vi "search house.vi"(8 "Nr Türen":i32, 9 "Häuser koord":i32[][](array[numeric])=[[160, 0], [220, 0], [220, 0], [280, 0], [280, 0], [340, 0], [20, 20], [80, 20], [190, 20], [250, 20], [310, 20], [220, 40], [280, 40], [50, 40], [120, 40], [160, 40], [220, 40], [280, 40], [340, 40], [340, 40], [160, 40], [380, 40], [20, 60], [80, 60], [140, 70], [360, 70], [160, 100], [380, 100], [120, 100], [120, 100], [180, 100], [240, 100], [340, 100], [380, 100], [280, 100], [320, 100], [20, 120], [60, 120], [150, 120], [350, 120], [260, 130], [180, 140], [120, 140], [320, 140], [320, 140], [380, 140], [360, 140], [40, 150], [280, 160], [240, 160], [340, 170], [20, 180], [60, 180], [45, 180], [5, 180], [360, 200], [160, 200], [320, 200], [120, 200], [25, 210], [200, 220], [240, 220], [140, 230], [5, 240], [0, 240], [45, 240], [60, 240], [220, 250], [120, 260], [30, 260], [130, 260], [160, 260], [190, 260], [60, 280], [200, 280], [240, 280], [0, 280], [160, 280], [300, 280], [360, 280], [240, 290], [200, 290], [130, 300], [190, 300], [330, 300], [220, 320], [300, 320], [360, 320], [300, 320], [360, 320], [330, 340], [200, 350], [240, 350], [300, 360], [360, 360], [30, 400], [90, 400], [60, 420], [30, 440], [90, 440]], 10 "Türen":string[][](array[string])=[["250", "40"], ["310", "40"], ["50", "60"], ["120", "70"], ["340", "70"], ["40", "120"], ["180", "120"], ["320", "120"], ["240", "130"], ["320", "170"], ["45", "210"], ["220", "220"], ["160", "230"], ["60", "260"], ["330", "280"], ["160", "300"], ["240", "320"], ["330", "360"], ["60", "400"], ["190", "40"]], 11 "Häuserlagen":cluster{i32[][]}[](array[cluster])=[{[[-30, 0], [30, 0], [30, -40], [-30, -40], [0, -20]]}, {[[0, 30], [0, -30], [-40, -30], [-40, 30], [-20, 0]]}, {[[30, 0], [-30, 0], [-30, 40], [30, 40], [0, 20]]}, {[[0, -30], [0, 30], [40, 30], [40, -30], [20, 0]]}, {[[0, 20], [60, 20], [60, -20], [0, -20], [30, 0]]}, {[[20, 0], [20, -60], [-20, -60], [-20, 0], [0, -30]]}, {[[0, -20], [-60, -20], [-60, 20], [0, 20], [-30, 0]]}, {[[-20, 0], [-20, 60], [20, 60], [20, 0], [0, 30]]}]) -> (3 "Häuser":T1[](array[typedef]))   [LabVIEW 2019]
uses:
  Haus.ctl
  Koordinate.ctl
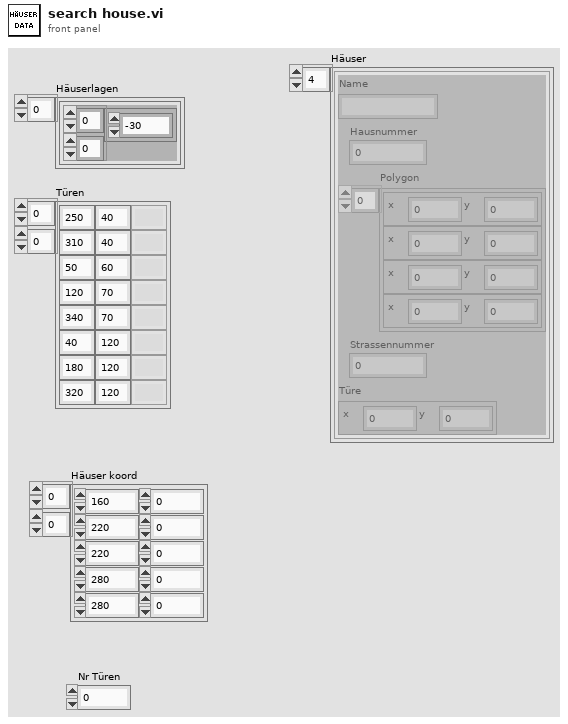
[diagram p1: front panel]
types:
  T1 = typedef "Haus.ctl" = cluster{"Name":string, "Hausnummer":u8, "Polygon":T2[], "Strassennummer":u8, "Türe":T2}
  T2 = typedef "Koordinate.ctl" = cluster{"x":dbl, "y":dbl}
  T3 = cluster{"Häuser koord[0]":i32, "Häuser koord[1]":i32}
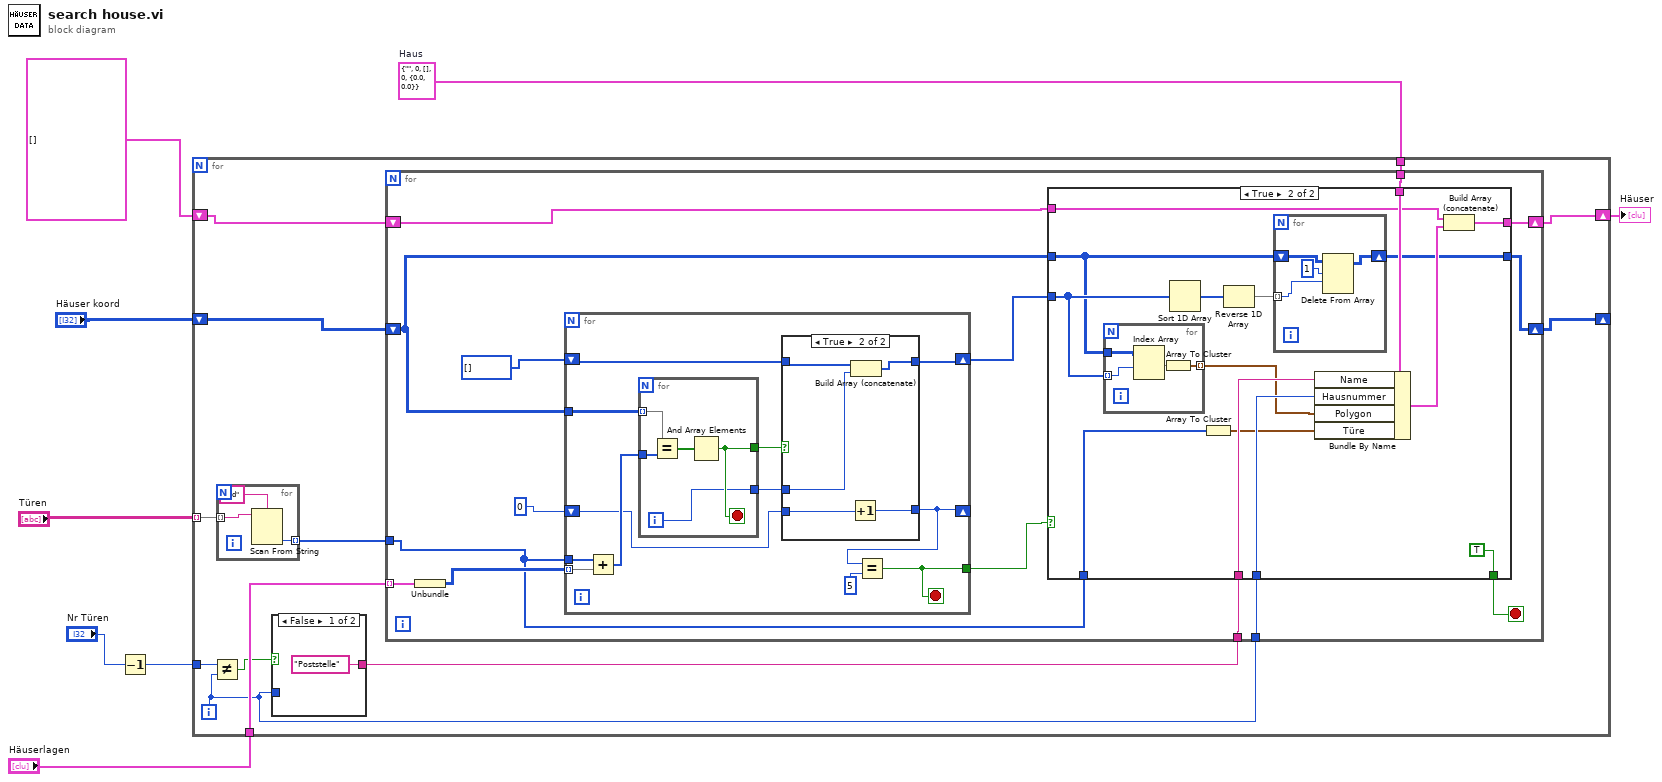
[diagram p0: block diagram]
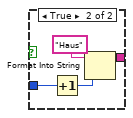
[diagram p2: hidden frame]
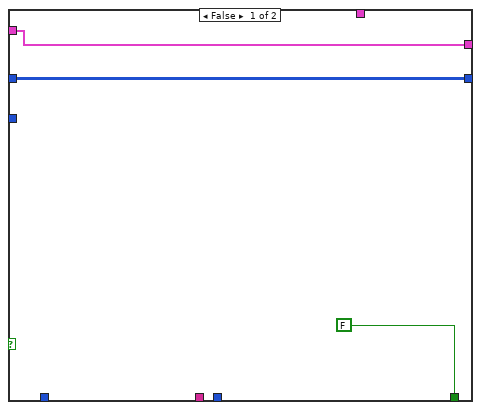
[diagram p4: hidden frame]
diagram:
  w5 = T1 {"Name"="", "Hausnummer"=0, "Polygon"=[], "Strassennummer"=0, "Türe"={"x"=0.0, "y"=0.0}}  # Haus
  n1 = Decrement(x="Nr Türen") -> (x-1=w1:i32)
  n2 = for {
    tunnel: "Türen" -> [w20] mode=indexing
    shift-right: [w13] -> _
    shift-left: "Häuser koord" -> [w18]
    tunnel: "Häuserlagen" -> [w19]
    shift-right: [w12] -> w4
    shift-left: T1[] [] -> [w15]
    tunnel: w5 -> [w16]
    tunnel: w1 -> [w11]
    i -> [w10]
    n3 = Not Equal?(x=w11, y=w10) -> (x != y?=w9:bool)
    n4 = for {
      tunnel: w20 -> [w93] mode=indexing
      tunnel: [w91] -> w17 mode=indexing
      n5 = Scan From String(format string="%d", input string=w93) -> (output 1=w91:i32)  [unwired: 3 in, 3 out]
    }
    n6 = case shown="False" w9 {
      tunnel: ["Poststelle" w25] -> w14
      tunnel: w10 -> [_ w23]
      frame False {
      }
      frame True {
        n7 = Increment(x=w23) -> (x+1=w24:i32)
        n8 = Format Into String(initial string="Haus", w24) -> (resulting string=w25:string)  [unwired: 2 in, 1 out]
      }
    }
    n9 = for {
      tunnel: w19 -> [w40] mode=indexing
      shift-right: [w27] -> w13
      shift-left: w18 -> [w28]
      tunnel: w17 -> [w38]
      tunnel: w16 -> [w37]
      shift-right: [w29] -> w12
      shift-left: w15 -> [w36]
      tunnel: w14 -> [w35]
      tunnel: w10 -> [w34]
      stop <- w31 stop-if-true
      n10 = Unbundle(w40) -> (w39:i32[][])
      n11 = for {
        tunnel: w39 -> [w52] mode=indexing
        tunnel: w38 -> [w49]
        shift-right: [w45] -> w30
        shift-left: i32[] [] -> [w47]
        shift-right: [w42] -> _
        shift-left: 0 -> [w46]
        tunnel: w28 -> [w51]
        tunnel: [w41] -> w26
        stop <- w41 stop-if-true
        n12 = Add(x=w49, y=w52) -> (x+y=w50:i32[])
        n13 = for {
          tunnel: w51 -> [w63] mode=indexing
          tunnel: w50 -> [w64]
          tunnel: [w61] -> w44
          tunnel: [w60] -> w48
          i -> [w60]
          stop <- w61 stop-if-true
          n14 = Equal?(x=w63, y=w64) -> (x = y?=w62:bool[])
          n15 = And Array Elements(Boolean array=w62) -> (logical AND=w61:bool)
        }
        n16 = case shown="True" w44 {
          tunnel: w46 -> [w54 w59]
          tunnel: [w54 w58] -> w42
          tunnel: [w53 w56] -> w45
          tunnel: w47 -> [w53 w57]
          tunnel: w48 -> [_ w55]
          frame False {
          }
          frame True {
            n17 = Increment(x=w59) -> (x+1=w58:i32)
            n18 = Build Array (concatenate)(w57, w55) -> (w56:i32[])
          }
        }
        n19 = Equal?(x=w42, y=5) -> (x = y?=w41:bool)
      }
      n20 = case shown="True" w26 {
        tunnel: w37 -> [_ w82]
        tunnel: w36 -> [w66 w76]
        tunnel: w35 -> [_ w81]
        tunnel: w34 -> [_ w80]
        tunnel: w38 -> [_ w79]
        tunnel: [FALSE TRUE] -> w31
        tunnel: w30 -> [_ w70]
        tunnel: [w66 w75] -> w29
        tunnel: w28 -> [w65 w69]
        tunnel: [w65 w71] -> w27
        frame False {
        }
        frame True {
          n21 = for {
            tunnel: w70 -> [w85] mode=indexing
            tunnel: w69 -> [w86]
            tunnel: [w83] -> w68 mode=indexing
            n22 = Index Array(array=w86, index (row)=w85) -> (element=w84:i32[])  [unwired: 1 in]
            n23 = Array To Cluster(array=w84) -> (cluster=w83:T3)
          }
          n24 = Sort 1D Array(array=w70) -> (sorted array=w73:i32[])
          n25 = Array To Cluster(array=w79) -> (cluster=w78:cluster{"[0]":i32, "[1]":i32})
          n26 = Reverse 1D Array(array=w73) -> (reversed array=w72:i32[])
          n27 = for {
            shift-right: [w89] -> w71
            shift-left: w69 -> [w90]
            tunnel: w72 -> [w88] mode=indexing
            n28 = Delete From Array(array=w90, length=1, index (row)=w88) -> (array with subset deleted=w89:i32[][])  [unwired: 1 in, 1 out]
          }
          n29 = Bundle By Name(cluster=w82, "Name"=w81, "Hausnummer"=w80, "Polygon"=w68, "Türe"=w78) -> (w74:T1)
          n30 = Build Array (concatenate)(w76, w74) -> (w75:T1[])
        }
      }
    }
  }
  "Häuser" <- w4
